vi "One Button Dialog with Timeout.vi"(1 "Btn Timeout(-1 s)":i32=-1, 2 "T button name (\"OK\")":string="OK", 3 "message":string) -> (0 "true":bool)   [LabVIEW 2017]
uses:
  a539abf7-d72e-4e1a-867b-c48a8ed28406.vi
panel:
  out "font":T1
  in  "btn":bool
  out "String":string
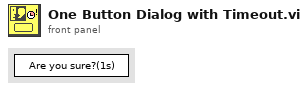
[diagram p1: front panel]
types:
  T1 = cluster{"Font Name:":string, "Size":i16, "Strikeout?":bool, "Italic?":bool, "Underline?":bool, "Outline?":bool, "Shadow?":bool, "Bold?":bool}
  T2 = typedef "LVFontTypeDef.ctl" = cluster{"Font Name":string, "Size":u16, "Bold":bool, "Italic":bool, "Underline":bool, "Strikeout":bool, "Color":u32}
  T3 = cluster{"left":i16, "top":i16, "right":i16, "bottom":i16}
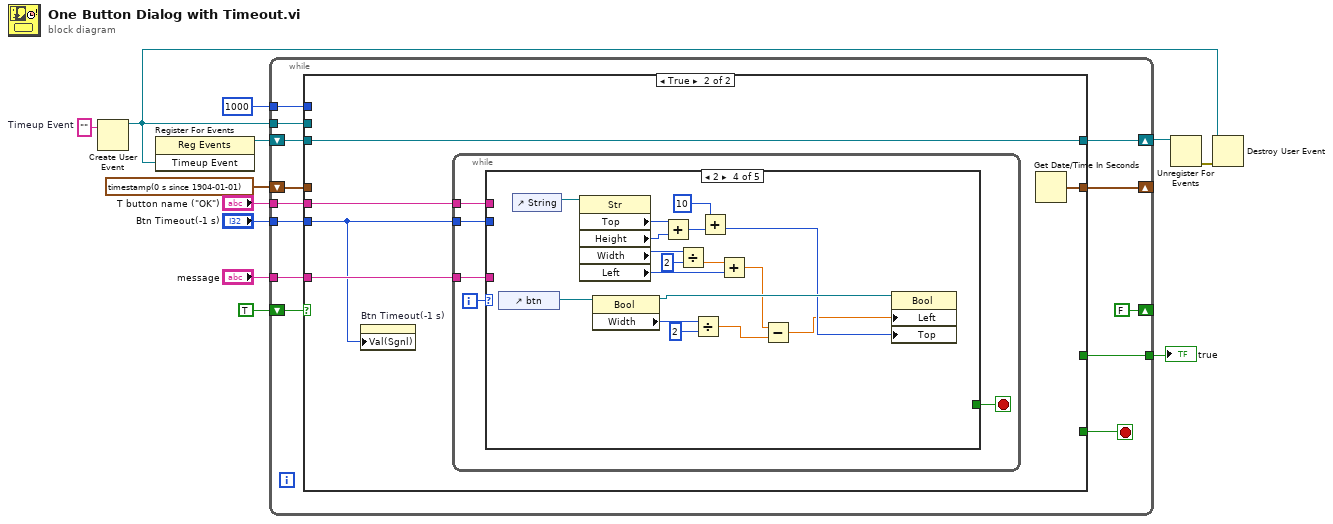
[diagram p0: block diagram]
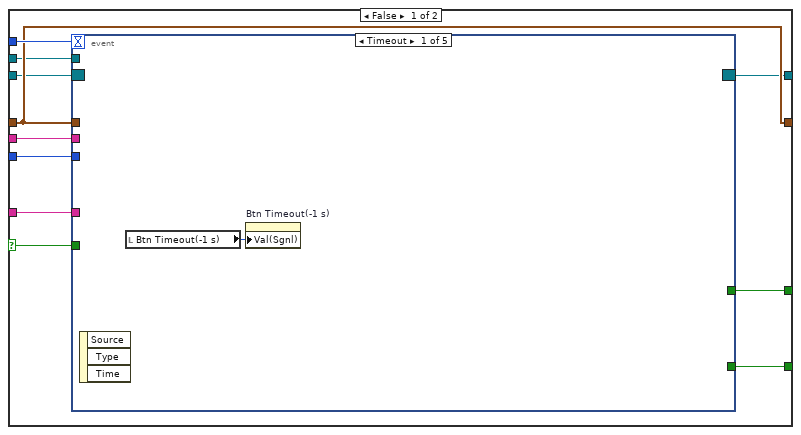
[diagram p2: hidden frame]
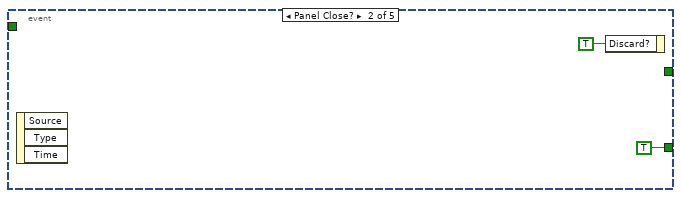
[diagram p3: hidden frame]
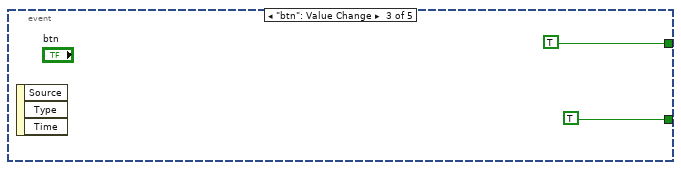
[diagram p4: hidden frame]
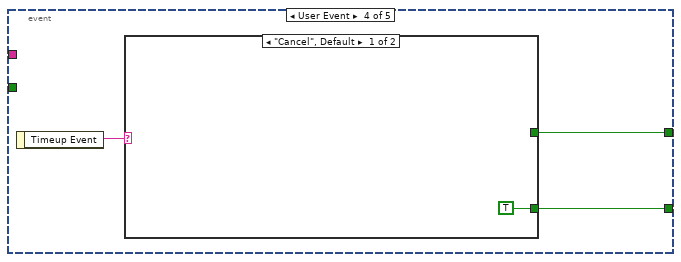
[diagram p5: hidden frame]
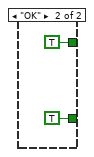
[diagram p6: hidden frame]
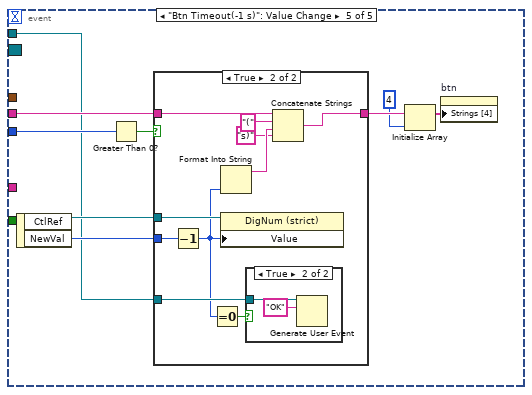
[diagram p7: hidden frame]
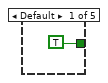
[diagram p10: hidden frame]
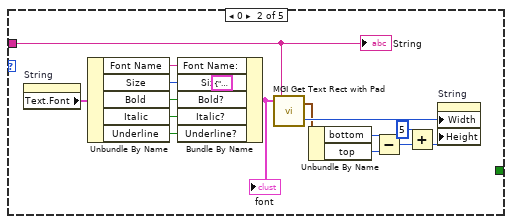
[diagram p11: hidden frame]
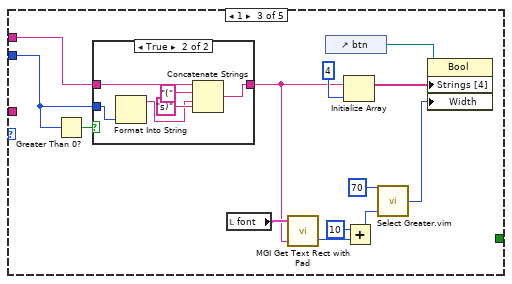
[diagram p12: hidden frame]
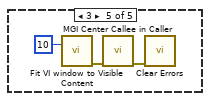
[diagram p14: hidden frame]
diagram:
  w5 = ""  # Timeup Event
  n1 = Create User Event(user event datatype=w5) -> (user event=w1:refnum<user-event>)  [unwired: 1 in, 1 out]
  n2 = register-events(w1) -> (reference out=w4:refnum<event-registration>)  [unwired: 2 in, 1 out]
  n3 = while {
    tunnel: [w24] -> w12
    tunnel: "T button name (\"OK\")" -> [w20]
    tunnel: "message" -> [w21]
    shift-right: [FALSE] -> _
    shift-left: TRUE -> [w23]
    tunnel: "Btn Timeout(-1 s)" -> [w19]
    shift-right: [w18] -> _
    shift-left: timestamp(0 s since 1904-01-01) ("seconds since 1Jan1904") -> [w17]
    tunnel: 1000 -> [w16]
    shift-right: [w14] -> w3
    shift-left: w4 -> [w15]
    tunnel: w1 -> [w13]
    stop <- w25 stop-if-true
    n4 = case shown="True" w23 {
      selector: w23 -> [w33 _]
      tunnel: [w36 _] -> w25
      tunnel: [w35 _] -> w24
      tunnel: w16 -> [w34 _]
      tunnel: w21 -> [w30 w72]
      tunnel: w20 -> [w32 w71]
      tunnel: w19 -> [w31 w70]
      tunnel: [w29 w74] -> w18
      tunnel: w17 -> [w29 _]
      tunnel: w15 -> [w28 w73]
      tunnel: [w27 w73] -> w14
      tunnel: w13 -> [w26 _]
      frame False {
        n5 = event shown="[0] Timeout" {
          selector: w28 -> [_ _ _ _ _]
          dyn-events: [_ _ _ _ _] -> w27
          timeout: w34 -> [_ _ _ _ _]
          tunnel: [_ TRUE ("Discard?") TRUE ("Discard?") w43 _] -> w36
          tunnel: [_ _ TRUE w42 _] -> w35
          tunnel: w33 -> [_ _ _ _ _]
          tunnel: w32 -> [_ _ _ _ w56]
          tunnel: w31 -> [_ _ _ _ w54]
          tunnel: w30 -> [_ _ _ _ _]
          tunnel: w29 -> [_ _ _ _ _]
          tunnel: w26 -> [_ _ _ _ w48]
          event Timeout {
            n6 = event-data() -> ()  [unwired: 1 in, 3 out]
            n7 = local read "Btn Timeout(-1 s)"() -> (w37:i32)
            n8 = property on="Btn Timeout(-1 s)" class="DigNum (strict)"("Val(Sgnl)"=w37) -> ()  [unwired: 2 in, 2 out]
          }
          event Panel Close? {
            n9 = event-data() -> ()  [unwired: 1 in, 3 out]
            n10 = event-data("Discard?"=TRUE) -> ()  [unwired: 1 in, 1 out]
          }
          event "btn": Value Change {
            n11 = event-data() -> ()  [unwired: 1 in, 3 out]
          }
          event User Event {
            n12 = event-data() -> ("Timeup Event"=w44:string)  [unwired: 1 in]
            n13 = case shown="\"Cancel\", Default" w44 {
              tunnel: [TRUE ("Discard?") TRUE ("Discard?")] -> w43
              tunnel: [_ TRUE ("Discard?")] -> w42
              frame "Cancel", Default {
              }
              frame "OK" {
              }
            }
          }
          event "Btn Timeout(-1 s)": Value Change {
            n14 = event-data() -> ("CtlRef"=w50:refnum<vi>, "NewVal"=w49:i32)  [unwired: 1 in]
            n15 = Greater Than 0?(x=w54) -> (x > 0?=w55:bool)
            n16 = case shown="True" w55 {
              tunnel: w56 -> [w57 w67]
              tunnel: [w57 w63] -> w53
              tunnel: w49 -> [_ w62]
              tunnel: w50 -> [_ w61]
              tunnel: w48 -> [_ w59]
              frame False {
              }
              frame True {
                n17 = Decrement(x=w62) -> (x-1=w58:i32)
                n18 = Equal To 0?(x=w58) -> (x = 0?=w60:bool)
                n19 = Format Into String(w58) -> (resulting string=w66:string)  [unwired: 3 in, 1 out]
                n20 = property class="DigNum (strict)"(reference=w61, "Value"=w58) -> ()  [unwired: 1 in, 2 out]
                n21 = case shown="True" w60 {
                  tunnel: w59 -> [_ w69]
                  frame False {
                  }
                  frame True {
                    n22 = Generate User Event(user event=w69, event data cluster="OK" ("event data")) -> ()  [unwired: 2 in, 2 out]
                  }
                }
                n23 = Concatenate Strings(w67, "(" ("string"), w66, "s)" ("string")) -> (w63:string)
              }
            }
            n24 = Initialize Array(w53, 4 ("dimension size")) -> (w52:string[])
            n25 = property on="btn" class="Bool"("Strings [4]"=w52) -> ()  [unwired: 2 in, 2 out]
          }
        }
      }
      frame True {
        n26 = property on="Btn Timeout(-1 s)" class="DigNum (strict)"("Val(Sgnl)"=w70) -> ()  [unwired: 2 in, 2 out]
        n27 = while {
          tunnel: w72 -> [w79]
          tunnel: w71 -> [w76]
          tunnel: w70 -> [w75]
          i -> [w78]
          stop <- w77 stop-if-true
          n28 = case shown="2" w78 {
            tunnel: w79 -> [_ w95 _ _ _]
            tunnel: [TRUE _ _ _ _] -> w77
            tunnel: w76 -> [_ _ w106 _ _]
            tunnel: w75 -> [_ _ w105 _ _]
            frame Default {
            }
            frame 0 {
              n29 = property on="String" class="Str"() -> ("Text.Font"=w96:T2)  [unwired: 2 in, 2 out]
              n30 = Unbundle By Name(w96) -> ("Font Name"=w92:string, "Size"=w91:u16, "Bold"=w90:bool, "Italic"=w88:bool, "Underline"=w89:bool)
              n31 = Bundle By Name(cluster=T1 {"Font Name:"="", "Size"=0, "Strikeout?"=FALSE, "Italic?"=FALSE, "Underline?"=FALSE, "Outline?"=FALSE, "Shadow?"=FALSE, "Bold?"=FALSE} ("Font"), "Font Name:"=w92, "Size"=w91, "Bold?"=w90, "Italic?"=w88, "Underline?"=w89) -> (w93:T1)
              "font" <- w93
              n32 = call <userlib>:"MGI Get Text Rect with Pad.vi"("Text"=w95, "Font"=w93) -> ("Width"=w87:i16, "Rect"=w86:T3)  [unwired: 1 in]
              n33 = Unbundle By Name(w86) -> ("bottom"=w83:i16, "top"=w85:i16)
              n34 = Subtract(x=w83, y=w85) -> (x-y=w84:i16)
              n35 = Add(x=i16 5, y=w84) -> (x+y=w82:i16)
              n36 = property on="String" class="Str"("Width"=w87, "Height"=w82) -> ()  [unwired: 2 in, 2 out]
              "String" <- w95
            }
            frame 1 {
              n37 = Greater Than 0?(x=w105) -> (x > 0?=w109:bool)
              n38 = case shown="True" w109 {
                tunnel: w106 -> [w110 w116]
                tunnel: [w110 w113] -> w102
                tunnel: w105 -> [_ w111]
                frame False {
                }
                frame True {
                  n39 = Format Into String(w111) -> (resulting string=w112:string)  [unwired: 3 in, 1 out]
                  n40 = Concatenate Strings(w116, "(" ("string"), w112, "s)" ("string")) -> (w113:string)
                }
              }
              n41 = local read "font"() -> (w103:T1)
              n42 = call <userlib>:"MGI Get Text Rect with Pad.vi"("Text"=w102, "Font"=w103) -> ("Width"=w101:i16)  [unwired: 1 in, 1 out]
              n43 = control-ref of="btn"() -> (w104:refnum<vi>)
              n44 = Initialize Array(w102, 4 ("dimension size")) -> (w108:string[])
              n45 = Add(x=i16 10, y=w101) -> (x+y=w98:i16)
              n46 = call "Select Greater.vim"("A"=70, "B"=w98) -> ("lesser"=w97:i32)  [unwired: 3 in]
              n47 = property on="Property Node" class="Bool"(reference=w104, "Strings [4]"=w108, "Width"=w97) -> ()  [unwired: 1 in, 2 out]
            }
            frame 2 {
              n48 = control-ref of="btn"() -> (w128:refnum<vi>)
              n49 = control-ref of="String"() -> (w133:refnum<vi>)
              n50 = property class="Str"(reference=w133) -> ("Top"=w132:i32, "Height"=w131:u32, "Width"=w123:u32, "Left"=w129:i32)  [unwired: 1 in, 2 out]
              n51 = property class="Bool"(reference=w128) -> (reference out=w127:refnum<vi>, "Width"=w121:u32)  [unwired: 1 in, 1 out]
              n52 = Add(x=w132, y=w131) -> (x+y=w130:u32)
              n53 = Divide(x=w123, y=u32 2) -> (x/y=w124:dbl)
              n54 = Divide(x=w121, y=u32 2) -> (x/y=w118:dbl)
              n55 = Add(x=u32 10, y=w130) -> (x+y=w126:u32)
              n56 = Add(x=w124, y=w129) -> (x+y=w119:dbl)
              n57 = Subtract(x=w119, y=w118) -> (x-y=w117:dbl)
              n58 = property class="Bool"(reference=w127, "Left"=w117, "Top"=w126) -> ()  [unwired: 1 in, 2 out]
            }
            frame 3 {
              n59 = call "Fit VI window to Visible Content.vi"("border spacing (2 px)"=10) -> ("error out"=w136:errorcluster)  [unwired: 5 in, 1 out]
              n60 = call <userlib>:"MGI Center Callee in Caller.vi"("Error In"=w136) -> ("Error Out"=w135:errorcluster)  [unwired: 10 in]
              n61 = call <vilib>:"Clear Errors.vi"("error in (no error)"=w135) -> ()  [unwired: 5 in, 2 out]
            }
          }
        }
        n62 = Get Date/Time In Seconds() -> (seconds since 1Jan1904=w74:timestamp)
      }
    }
  }
  "true" <- w12
  n63 = Unregister For Events(event registration refnum=w3) -> (error out=w2:errorcluster)  [unwired: 1 in]
  n64 = Destroy User Event(user event=w1, error in=w2) -> ()  [unwired: 1 out]
